vi "Generate Timestamped Filepath.vi"(8 "Error In":errorcluster, 10 "appended filename":string) -> (0 "Error Out":errorcluster, 3 "timestamped relative filepath":path)   [LabVIEW 2020]
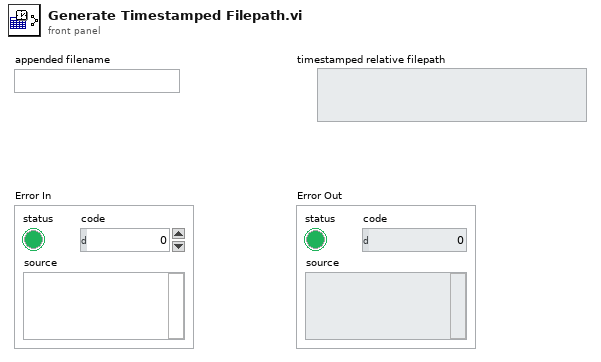
[diagram p1: front panel]
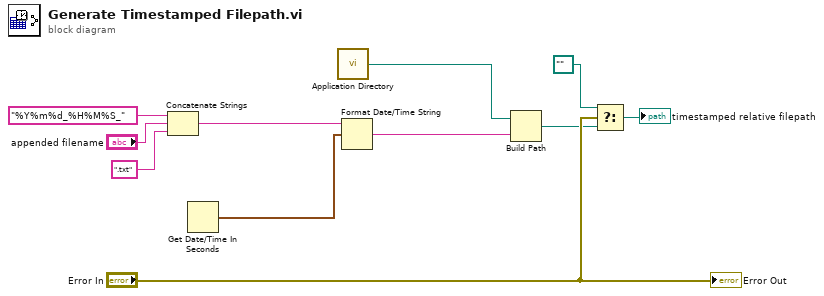
[diagram p0: block diagram]
diagram:
  n1 = Concatenate Strings "Concatenate Strings"("%Y%m%d_%H%M%S_" ("string"), "appended filename", ".txt" ("string")) -> (w7:string)
  n2 = Get Date/Time In Seconds() -> (seconds since 1Jan1904=w8:timestamp)
  n3 = call <vilib>:"Application Directory.vi"() -> ("Application Directory"=w6:path)
  n4 = Format Date/Time String(time format string (%c)=w7, seconds (now)=w8) -> (date/time string=w5:string)  [unwired: 1 in]
  n5 = Build Path(base path=w6, name or relative path=w5) -> (appended path=w3:path)
  n6 = Select(t=path "", s="Error In", f=w3) -> (s? t:f=→"timestamped relative filepath":path)
  "Error Out" <- "Error In"
